vi "_Write.vi"(8 "error in (no error)":errorcluster, 9 "Message":string, 10 "Level":T1, 11 "Name":T2) -> (0 "error out":errorcluster)   [LabVIEW 2023, in "Log.lvclass"]
uses:
  Log.lvclass
  Log_Facilities.ctl
  Log_Level.ctl
  Log_Facility.ctl
  Helpers/UTC.ctl
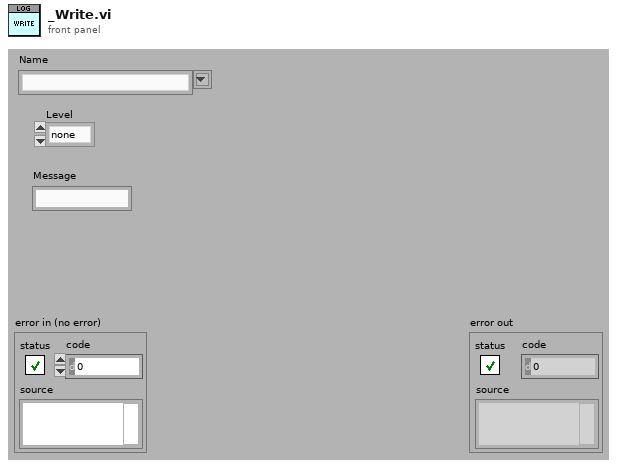
[diagram p1: front panel]
types:
  T1 = typedef "Log.lvclass/Log_Level.ctl" = enum16{"none", "info", "trace", "warn", "error", "fatal"}
  T2 = typedef "Log.lvclass/Log_Facilities.ctl" = string
  T3 = typedef "Log.lvclass/Log_Facility.ctl" = cluster{"Path":path, "Ref":refnum<file>, "Level":T1}
  T4 = typedef "UTC.ctl" = string
  T5 = typedef "Log.lvclass/ObjectAttributes.ctl" = cluster{"Level":T1, "Facilities":variant, "Event":refnum<user-event>}
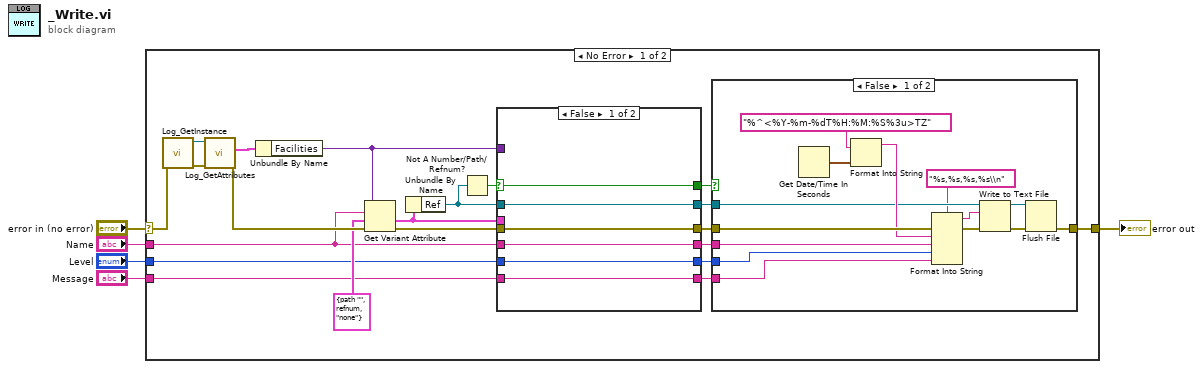
[diagram p0: block diagram]
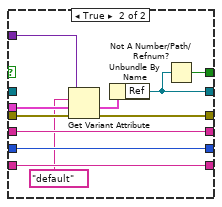
[diagram p2: hidden frame]
diagram:
  n1 = case shown="No Error" "error in (no error)" {
    selector: "error in (no error)" -> [w26 w59]
    tunnel: [w22 w59] -> w4
    tunnel: "Name" -> [w13 _]
    tunnel: "Level" -> [w12 _]
    tunnel: "Message" -> [w11 _]
    frame No Error {
      n2 = call "Log_GetInstance.vi"("error in (no error)"=w26) -> ("error out"=w25:errorcluster, "reference out"=w21:refnum<class "Log.lvclass">)  [unwired: 6 in, 3 out]
      n3 = call "Log_GetAttributes.vi"("error in (no error)"=w25, "reference in"=w21) -> ("error out"=w24:errorcluster, "Data"=w20:T5)  [unwired: 6 in, 2 out]
      n4 = Unbundle By Name(w20) -> ("Facilities"=w18:variant)
      n5 = Get Variant Attribute(Variant=w18, name=w13, default value (empty Variant)=T3 {"Path"=path "", "Ref"=refnum, "Level"=enum."none"} ("Cluster"), error in=w24) -> (value=w7:T3, error out=w17:errorcluster)  [unwired: 2 out]
      n6 = Unbundle By Name(w7) -> ("Ref"=w16:refnum<file>)
      n7 = Not A Number/Path/Refnum?(number/path/refnum=w16) -> (NaN/Path/Refnum?=w19:bool)
      n8 = case shown="False" w19 {
        selector: w19 -> [w27 _]
        tunnel: w18 -> [_ w42]
        tunnel: w17 -> [w31 w41]
        tunnel: w16 -> [w32 _]
        tunnel: [w32 w35] -> w15
        tunnel: [w31 w36] -> w14
        tunnel: w13 -> [w30 w38]
        tunnel: w12 -> [w29 w39]
        tunnel: w11 -> [w28 w40]
        tunnel: [w30 w38] -> w10
        tunnel: [w29 w39] -> w9
        tunnel: [w28 w40] -> w8
        tunnel: w7 -> [_ w37]
        tunnel: [w27 w34] -> w6
        frame False {
        }
        frame True {
          n9 = Get Variant Attribute(Variant=w42, name=T2 "default" ("Facility (default)"), default value (empty Variant)=w37, error in=w41) -> (value=w43:T3, error out=w36:errorcluster)  [unwired: 2 out]
          n10 = Unbundle By Name(w43) -> ("Ref"=w35:refnum<file>)
          n11 = Not A Number/Path/Refnum?(number/path/refnum=w35) -> (NaN/Path/Refnum?=w34:bool)
        }
      }
      n12 = case shown="False" w6 {
        tunnel: w14 -> [w57 w58]
        tunnel: w10 -> [w56 _]
        tunnel: w9 -> [w55 _]
        tunnel: w8 -> [w54 _]
        tunnel: w15 -> [w48 _]
        tunnel: [w46 w58] -> w22
        frame False {
          n13 = Get Date/Time In Seconds() -> (seconds since 1Jan1904=w52:timestamp)
          n14 = Format Into String(format string=T4 "%^<%Y-%m-%dT%H:%M:%S%3u>TZ" ("UTC"), w52) -> (resulting string=w51:string)  [unwired: 2 in, 1 out]
          n15 = Format Into String(format string="%s,%s,%s,%s\\n", error in=w57, w51, w56, w55, w54) -> (resulting string=w49:string, error out=w50:errorcluster)  [unwired: 1 in]
          n16 = Write to Text File(file (use dialog)=w48, text=w49, error in=w50) -> (refnum out=w45:refnum<file>, error out=w47:errorcluster)  [unwired: 1 in, 1 out]
          n17 = Flush File(refnum=w45, error in=w47) -> (error out=w46:errorcluster)  [unwired: 1 out]
        }
        frame True {
        }
      }
    }
    frame Error {
    }
  }
  "error out" <- w4
